vi "светофор.vi"() -> ()   [LabVIEW 2019]
panel:
  in  "...":bool
  out "red":bool
  out "Numeric":dbl
  in  "stop":bool
  out "green":bool
  out "yellow":bool
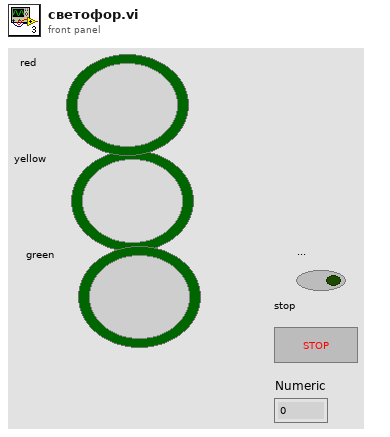
[diagram p1: front panel]
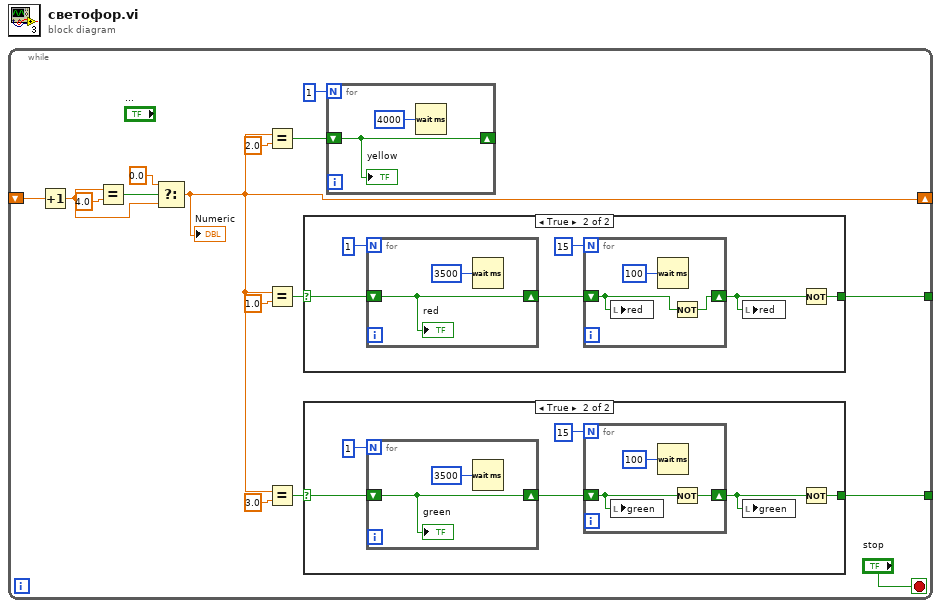
[diagram p0: block diagram]
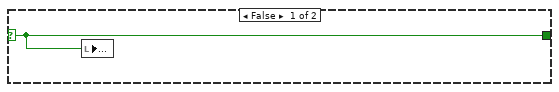
[diagram p2: hidden frame]
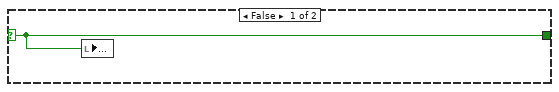
[diagram p3: hidden frame]
diagram:
  n1 = while {
    shift-right: [w8] -> _
    shift-left: _ -> [w13]
    tunnel: [w4] -> _
    tunnel: [w3] -> _
    stop <- "stop" stop-if-true
    n2 = Increment(x=w13) -> (x+1=w10:dbl)
    n3 = Equal?(x=w10, y=4.0 ("x")) -> (x = y?=w12:bool)
    n4 = Select(t=0.0, s=w12, f=w10) -> (s? t:f=w8:dbl)
    "Numeric" <- w8
    n5 = Equal?(x=w8, y=2.0) -> (x = y?=w1:bool)
    n6 = Equal?(x=w8, y=1.0) -> (x = y?=w5:bool)
    n7 = Equal?(x=w8, y=3.0) -> (x = y?=w6:bool)
    n8 = case shown="True" w5 {
      selector: w5 -> [w31 w34]
      tunnel: [w31 w33] -> w4
      frame False {
        n9 = local write "..."(w31) -> ()
      }
      frame True {
        n10 = for {
          N: 1 -> [_]
          shift-right: [w38] -> w35
          shift-left: w34 -> [w38]
          n11 = Wait (ms)(milliseconds to wait=u32 3500 ("millisecond timer value")) -> ()  [unwired: 1 out]
          "red" <- w38
        }
        n12 = for {
          N: 15 -> [_]
          shift-right: [w41] -> w32
          shift-left: w35 -> [w40]
          n13 = local write "red"(w40) -> ()
          n14 = Wait (ms)(milliseconds to wait=100) -> ()  [unwired: 1 out]
          n15 = Not(x=w40) -> (.not. x?=w41:bool)
        }
        n16 = local write "red"(w32) -> ()
        n17 = Not(x=w32) -> (.not. x?=w33:bool)
      }
    }
    n18 = case shown="True" w6 {
      selector: w6 -> [w19 w22]
      tunnel: [w19 w21] -> w3
      frame False {
        n19 = local write "..."(w19) -> ()
      }
      frame True {
        n20 = for {
          N: 1 -> [_]
          shift-right: [w27] -> w24
          shift-left: w22 -> [w27]
          n21 = Wait (ms)(milliseconds to wait=u32 3500 ("millisecond timer value")) -> ()  [unwired: 1 out]
          "green" <- w27
        }
        n22 = for {
          N: 15 -> [_]
          shift-right: [w29] -> w20
          shift-left: w24 -> [w28]
          n23 = local write "green"(w28) -> ()
          n24 = Wait (ms)(milliseconds to wait=100) -> ()  [unwired: 1 out]
          n25 = Not(x=w28) -> (.not. x?=w29:bool)
        }
        n26 = local write "green"(w20) -> ()
        n27 = Not(x=w20) -> (.not. x?=w21:bool)
      }
    }
    n28 = for {
      N: 1 -> [_]
      shift-right: [w18] -> _
      shift-left: w1 -> [w18]
      n29 = Wait (ms)(milliseconds to wait=u32 4000 ("millisecond timer value")) -> ()  [unwired: 1 out]
      "yellow" <- w18
    }
  }
